vi "test-quintic-spline-05.vi"() -> (3 "Test Passed":bool)   [LabVIEW 2019]
uses:
  <vilib>/Rock Robotics/WPI/ThirdParty/JAS_Junk/TrajLib/POSEwCURVATURE.ctl
  <vilib>/Rock Robotics/WPI/ThirdParty/JAS_Junk/TrajLib/POSE2D.ctl
  <vilib>/Rock Robotics/WPI/ThirdParty/JAS_Junk/TrajLib/TRANSLATION2D.ctl
  <vilib>/Rock Robotics/WPI/ThirdParty/JAS_Junk/TrajLib/ROTATION2D.ctl
  <vilib>/Rock Robotics/WPI/ThirdParty/JAS_Junk/TrajLib/Rotation2d_CreateAngle.vi
  <vilib>/Rock Robotics/WPI/ThirdParty/JAS_Junk/TrajLib/Translation2d_Create.vi
  <vilib>/Rock Robotics/WPI/ThirdParty/JAS_Junk/TrajLib/Util_CalcDist.vi
  <vilib>/Rock Robotics/WPI/ThirdParty/JAS_Junk/TrajLib/Trajectory_Library.lvlib
panel:
  out "XY Graph":cluster{dbl[], dbl[]}(graph)
  out "Numb\nWaypoints":i32
  out "All Interior \nwayPoints\nFound (True)":bool
  out "end rot = 0":dbl
  out "end y = 0":dbl
  out "end x = 0":dbl
  out "start rot = 0":dbl
  out "start y = 0":dbl
  out "start x = 0":dbl
  out "max dtheta < 0.0872":dbl
  out "max dy < 0.00127":dbl
  out "max dx  < 0.127":dbl
  out "Overall Error":errorcluster
  out "Elements":i32
  out "Create Spline Error":errorcluster
  out "SplinePoses\nWCurve":T1[](array[typedef]) {"POSE"."ROTATION"."SIN" format="%13.4f"; "POSE"."ROTATION"."COS" format="%13.4f"; "POSE"."ROTATION"."VALUE" format="%13.4f"; "POSE"."TRANSLATION"."Y" format="%14.3f"; "POSE"."TRANSLATION"."X" format="%14.3f"}
  out "Elapsed Time":dbl
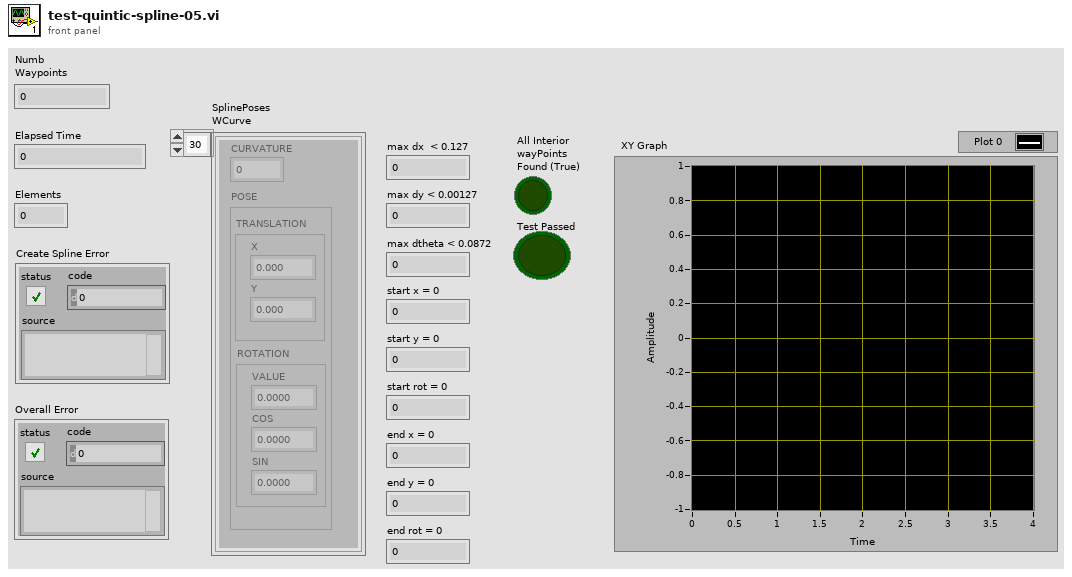
[diagram p1: front panel]
types:
  T1 = typedef "Trajectory_Library.lvlib/POSEwCURVATURE.ctl" = cluster{"CURVATURE":dbl, "POSE":T2}
  T2 = typedef "Trajectory_Library.lvlib/POSE2D.ctl" = cluster{"TRANSLATION":T3, "ROTATION":T4}
  T3 = typedef "Trajectory_Library.lvlib/TRANSLATION2D.ctl" = cluster{"X":dbl, "Y":dbl}
  T4 = typedef "Trajectory_Library.lvlib/ROTATION2D.ctl" = cluster{"VALUE":dbl, "COS":dbl, "SIN":dbl}
  T5 = typedef "Trajectory_Library.lvlib/SPLINE.ctl" = cluster{"Degree":i32, "Coefficients":T6}
  T6 = typedef "NI_Matrix.lvlib/RealMatrix.ctl" = dbl[][]
  T7 = typedef "Trajectory_Library.lvlib/TWIST2D.ctl" = cluster{"dX":dbl, "dY":dbl, "dTHETA":dbl}
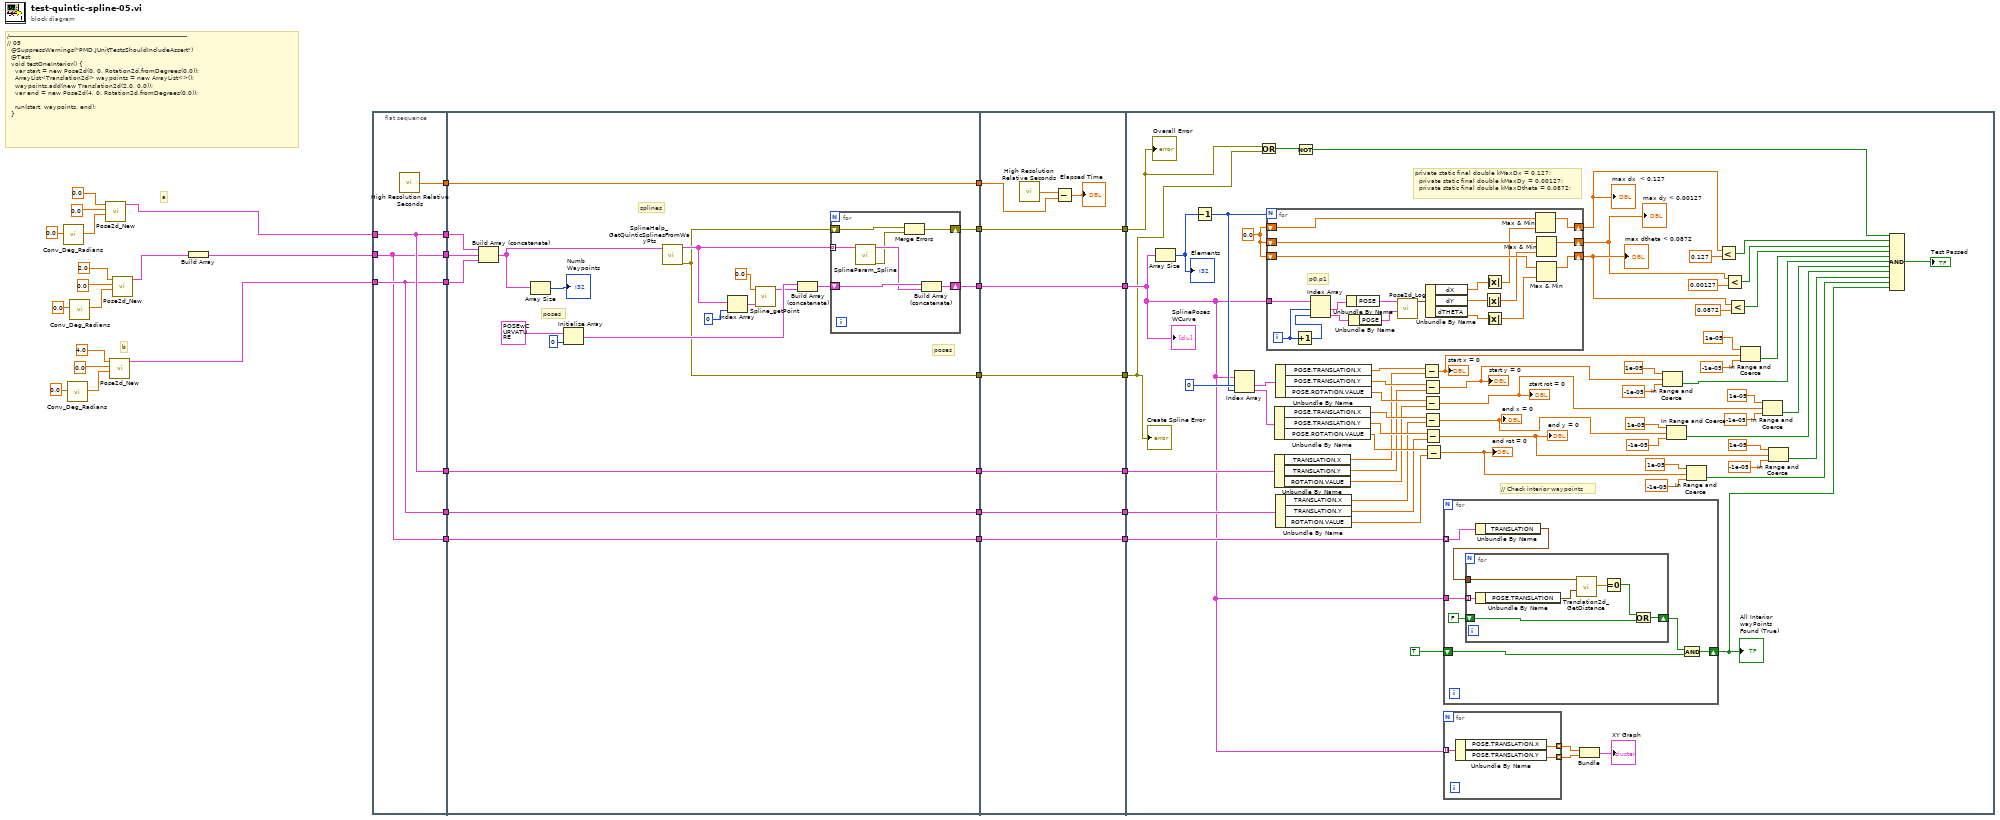
[diagram p0: block diagram]
diagram:
  # "b"
  # "a"
  # "/-----------------------------------------------------------------------------------------\n// 05\n  @SuppressWarnings(\"PMD.JUnitTestsShouldIncludeAssert\")\n  @Test\n  void testOneInterior() {\n    var start = new Pose2d(0, 0, Rotation2d.fromDegrees(0.0));\n    ArrayList<Translation2d> waypoints = new ArrayList<>();\n    waypoints.add(new Translation2d(2.0, 0.0));\n    var end = new Pose2d(4, 0, Rotation2d.fromDegrees(0.0));\n\n    run(start, waypoints, end);\n  }"
  n1 = call <vilib>:"Conv_Deg_Radians.vi"("Degress"=0.0) -> ("Radians"=w11:dbl)  [unwired: 10 in]
  n2 = call <vilib>:"Conv_Deg_Radians.vi"("Degress"=0.0) -> ("Radians"=w14:dbl)  [unwired: 10 in]
  n3 = call <vilib>:"Conv_Deg_Radians.vi"("Degress"=0.0) -> ("Radians"=w6:dbl)  [unwired: 10 in]
  n4 = call <vilib>:"Pose2d_New.vi"("Heading"=w11, "Y"=0.0, "X"=0.0) -> ("out POSe"=w2:T2)  [unwired: 8 in]
  n5 = call <vilib>:"Pose2d_New.vi"("Heading"=w14, "Y"=0.0, "X"=4.0) -> ("out POSe"=w1:T2)  [unwired: 8 in]
  n6 = call <vilib>:"Pose2d_New.vi"("Heading"=w6, "Y"=0.0, "X"=2.0) -> ("out POSe"=w4:T2)  [unwired: 8 in]
  n7 = Build Array(w4) -> (w3:T2[])
  n8 = flat-sequence {
    tunnel: w2 -> [w39]
    tunnel: [w39] -> w36
    tunnel: w1 -> [w38]
    tunnel: [w38] -> w35
    tunnel: [w40] -> w34
    tunnel: [w39] -> w26
    tunnel: [w38] -> w23
    tunnel: [w37] -> w18
    tunnel: w3 -> [w37]
    tunnel: [w37] -> w17
    tunnel: w36 -> [w45]
    tunnel: w35 -> [w44]
    tunnel: [w61] -> w33
    tunnel: w34 -> [w61]
    tunnel: [w51] -> w32
    tunnel: [w50] -> w30
    tunnel: [w49] -> w28
    tunnel: w26 -> [w48]
    tunnel: [w48] -> w25
    tunnel: w23 -> [w47]
    tunnel: [w47] -> w22
    tunnel: [w46] -> w19
    tunnel: w18 -> [w46]
    tunnel: w17 -> [w42]
    tunnel: w33 -> [w77]
    tunnel: w32 -> [w76]
    tunnel: [w76] -> w31
    tunnel: w30 -> [w75]
    tunnel: [w75] -> w29
    tunnel: w28 -> [w74]
    tunnel: [w74] -> w27
    tunnel: w25 -> [w71]
    tunnel: [w71] -> w24
    tunnel: w22 -> [w70]
    tunnel: [w70] -> w21
    tunnel: [w69] -> w20
    tunnel: w19 -> [w69]
    tunnel: w31 -> [w118]
    tunnel: w29 -> [w106]
    tunnel: w27 -> [w105]
    tunnel: w24 -> [w140]
    tunnel: w21 -> [w139]
    tunnel: w20 -> [w122]
    frame #0 {
      n9 = call <vilib>:"High Resolution Relative Seconds.vi"() -> ("relative seconds"=w40:dbl)
    }
    frame #1 {
      # "poses"
      # "poses"
      # "splines"
      n10 = Build Array (concatenate)(w45, w42, w44) -> (w41:T2[])
      n11 = Array Size(array=w41) -> (size(s)=→"Numb\nWaypoints":i32)
      n12 = Initialize Array(T1 {"CURVATURE"=0.0, "POSE"={"TRANSLATION"={"X"=0.0, "Y"=0.0}, "ROTATION"={"VALUE"=0.0, "COS"=1.0, "SIN"=0.0}}} ("POSEwCURVATURE"), 0 ("dimension size")) -> (w55:T1[])
      n13 = call <vilib>:"SplineHelp_GetQuinticSplinesFromWayPts.vi"("WayPoints"=w41) -> ("out Error"=w50:errorcluster, "Splines"=w52:T5[])  [unwired: 9 in]
      n14 = Index Array(array=w52, index=0) -> (element=w57:T5)
      n15 = call <vilib>:"Spline_getPoint.vi"("inputSPLINE"=w57, "Time"=0.0) -> ("POSEwCURVATURE"=w54:T1)  [unwired: 9 in]
      n16 = Build Array (concatenate)(w55, w54) -> (w53:T1[])
      n17 = for {
        shift-right: [w65] -> w51
        shift-left: w53 -> [w67]
        tunnel: w52 -> [w68] mode=indexing
        shift-right: [w63] -> w49
        shift-left: w50 -> [w64]
        n18 = call <vilib>:"SplineParam_Spline.vi"("inputSPLINE"=w68) -> ("error out"=w62:errorcluster, "outputPOSEwCURVATURE"=w66:T1[])  [unwired: 9 in]
        n19 = Merge Errors(w64, w62) -> (w63:errorcluster)
        n20 = Build Array (concatenate)(w67, w66) -> (w65:T1[])
      }
    }
    frame #2 {
      n21 = call <vilib>:"High Resolution Relative Seconds.vi"() -> ("relative seconds"=w72:dbl)
      n22 = Subtract(x=w72, y=w77) -> (x-y=→"Elapsed Time":dbl)
    }
    frame #3 {
      w141 = 0.0
      # "// Check interior waypoints"
      # "private static final double kMaxDx = 0.127;\n  private static final double kMaxDy = 0.00127;\n  private static final double kMaxDtheta = 0.0872;"
      n23 = Array Size(array=w118) -> (size(s)=w142:i32)
      "Elements" <- w142
      n24 = Decrement(x=w142) -> (x-1=w137:i32)
      n25 = Index Array(array=w118, index #1=0 ("index"), index #2=w137) -> (element #1=w136:T1, element #2=w135:T1)
      n26 = Or(x=w105, y=w106) -> (x .or. y?=w107:bool)
      n27 = for {
        N: w137 -> [_]
        tunnel: w118 -> [w177]
        shift-right: [w168] -> w111
        shift-left: w141 -> [w165]
        shift-right: [w166] -> w113
        shift-left: w141 -> [w163]
        shift-right: [w167] -> w112
        shift-left: w141 -> [w164]
        i -> [w179]
        # "p0,p1"
        n28 = Increment(x=w179) -> (x+1=w178:i32)
        n29 = Index Array(array=w177, index #1=w179, index #2=w178) -> (element #1=w176:T1, element #2=w175:T1)
        n30 = Unbundle By Name(w176) -> ("POSE"=w174:T2)
        n31 = Unbundle By Name(w175) -> ("POSE"=w173:T2)
        n32 = call <vilib>:"Pose2d_Log.vi"("end POSE"=w173, "in POSE"=w174) -> ("out TWIST"=w172:T7)  [unwired: 9 in]
        n33 = Unbundle By Name(w172) -> ("dX"=w169:dbl, "dY"=w170:dbl, "dTHETA"=w171:dbl)
        n34 = Absolute Value(x=w170) -> (abs(x)=w161:dbl)
        n35 = Absolute Value(x=w169) -> (abs(x)=w162:dbl)
        n36 = Absolute Value(x=w171) -> (abs(x)=w160:dbl)
        n37 = Max & Min(x=w165, y=w162) -> (max(x,y)=w168:dbl)  [unwired: 1 out]
        n38 = Max & Min(x=w164, y=w161) -> (max(x,y)=w167:dbl)  [unwired: 1 out]
        n39 = Max & Min(x=w163, y=w160) -> (max(x,y)=w166:dbl)  [unwired: 1 out]
      }
      "max dx  < 0.127" <- w111
      "max dy < 0.00127" <- w112
      "max dtheta < 0.0872" <- w113
      n40 = Unbundle By Name(w135) -> ("POSE.TRANSLATION.X"=w131:dbl, "POSE.TRANSLATION.Y"=w130:dbl, "POSE.ROTATION.VALUE"=w129:dbl)
      n41 = Unbundle By Name(w140) -> ("TRANSLATION.X"=w128:dbl, "TRANSLATION.Y"=w127:dbl, "ROTATION.VALUE"=w126:dbl)
      n42 = Unbundle By Name(w136) -> ("POSE.TRANSLATION.X"=w134:dbl, "POSE.TRANSLATION.Y"=w133:dbl, "POSE.ROTATION.VALUE"=w132:dbl)
      n43 = Unbundle By Name(w139) -> ("TRANSLATION.X"=w125:dbl, "TRANSLATION.Y"=w124:dbl, "ROTATION.VALUE"=w123:dbl)
      n44 = Not(x=w107) -> (.not. x?=w104:bool)
      n45 = Subtract(x=w134, y=w128) -> (x-y=w100:dbl)
      "start x = 0" <- w100
      n46 = Subtract(x=w133, y=w127) -> (x-y=w79:dbl)
      "start y = 0" <- w79
      n47 = Subtract(x=w132, y=w126) -> (x-y=w83:dbl)
      "start rot = 0" <- w83
      n48 = Subtract(x=w131, y=w125) -> (x-y=w84:dbl)
      "end x = 0" <- w84
      n49 = Subtract(x=w130, y=w124) -> (x-y=w91:dbl)
      "end y = 0" <- w91
      n50 = Subtract(x=w129, y=w123) -> (x-y=w95:dbl)
      "end rot = 0" <- w95
      n51 = for {
        tunnel: w122 -> [w147] mode=indexing
        tunnel: w118 -> [w152]
        shift-right: [w151] -> w103
        shift-left: TRUE -> [w150]
        n52 = Unbundle By Name(w147) -> ("TRANSLATION"=w146:T3)
        n53 = for {
          tunnel: w152 -> [w156] mode=indexing
          shift-right: [w159] -> w148
          shift-left: FALSE -> [w158]
          tunnel: w146 -> [w157]
          n54 = Unbundle By Name(w156) -> ("POSE.TRANSLATION"=w155:T3)
          n55 = call <vilib>:"Translation2d_GetDistance.vi"("other Translation"=w155, "In Translation"=w157) -> ("Distance"=w154:dbl)  [unwired: 9 in]
          n56 = Equal To 0?(x=w154) -> (x = 0?=w153:bool)
          n57 = Or(x=w153, y=w158) -> (x .or. y?=w159:bool)
        }
        n58 = And(x=w148, y=w150) -> (x .and. y?=w151:bool)
      }
      "All Interior \nwayPoints\nFound (True)" <- w103
      n59 = for {
        tunnel: [w145] -> w120 mode=indexing
        tunnel: [w144] -> w119 mode=indexing
        tunnel: w118 -> [w143] mode=indexing
        n60 = Unbundle By Name(w143) -> ("POSE.TRANSLATION.X"=w145:dbl, "POSE.TRANSLATION.Y"=w144:dbl)
      }
      n61 = Bundle(w120, w119) -> (→"XY Graph":cluster{dbl[], dbl[]})  [unwired: 1 in]
      n62 = In Range and Coerce(upper limit=1e-05, x=w79, lower limit=-1e-05) -> (In Range?=w80:bool)  [unwired: 1 out]
      n63 = In Range and Coerce(upper limit=1e-05, x=w84, lower limit=-1e-05) -> (In Range?=w86:bool)  [unwired: 1 out]
      n64 = In Range and Coerce(upper limit=1e-05, x=w95, lower limit=-1e-05) -> (In Range?=w96:bool)  [unwired: 1 out]
      n65 = Less?(x=w111, y=0.127) -> (x < y?=w110:bool)
      n66 = Less?(x=w112, y=0.00127) -> (x < y?=w109:bool)
      n67 = Less?(x=w113, y=0.0872) -> (x < y?=w108:bool)
      n68 = In Range and Coerce(upper limit=1e-05, x=w100, lower limit=-1e-05) -> (In Range?=w99:bool)  [unwired: 1 out]
      n69 = In Range and Coerce(upper limit=1e-05, x=w83, lower limit=-1e-05) -> (In Range?=w85:bool)  [unwired: 1 out]
      n70 = In Range and Coerce(upper limit=1e-05, x=w91, lower limit=-1e-05) -> (In Range?=w92:bool)  [unwired: 1 out]
      n71 = Compound Arithmetic op=AND(w104, w110, w109, w108, w99, w80, w85, w86, w92, w96, w103) -> (→"Test Passed":bool)
      "SplinePoses\nWCurve" <- w118
      "Create Spline Error" <- w106
      "Overall Error" <- w105
    }
  }
